vi "GetText.vi"(8 "error in":errorcluster, 11 "Systems in":refnum<class "Systems.lvclass">) -> (0 "error out":errorcluster, 1 "additional text":string, 2 "text":string, 3 "Systems out":refnum<class "Systems.lvclass">, 4 "glyph":string)   [LabVIEW 2013, in "PL Framework Configuration Tool.lvlib" / "Systems.lvclass"]
uses:
  Systems.lvclass
  subVIs/Glyphs Status.ctl
  TBM Configuration Node/TBM Configuration Node.lvclass
  PL Framework Configuration Tool.lvlib
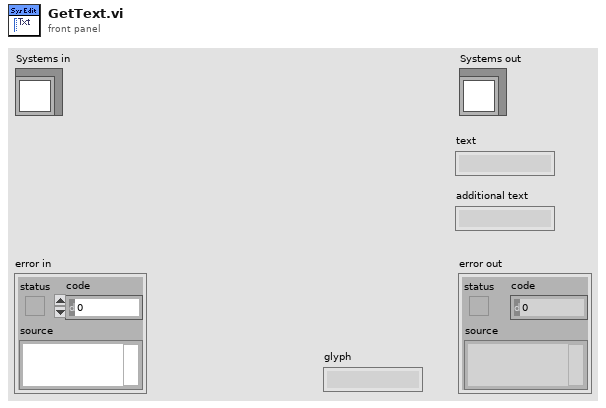
[diagram p1: front panel]
types:
  T1 = typedef "PL Framework Configuration Tool.lvlib/Glyphs Status.ctl" = enum16{"Normal", "Error"}
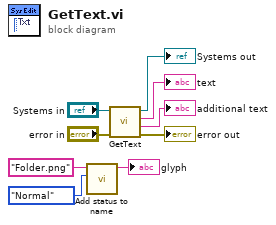
[diagram p0: block diagram]
diagram:
  n1 = call "Add status to name.vi"("Status"=Glyphs_Status."Normal", "Name"="Folder.png" ("glyph")) -> ("Name with status"=→"glyph":string)  [unwired: 9 in]
  n2 = call-parent "GetText.vi"("error in"="error in", "node in"="Systems in") -> ("error out"=→"error out":errorcluster, "additional text"=→"additional text":string, "text"=→"text":string, "node out"=→"Systems out":refnum<class "Systems.lvclass">)  [unwired: 5 in, 1 out]
